vi "Determine Actions.vi"(8 "View":i32[](array[numeric]) caption="View (Team Index, -1: empty)", 9 "Team Index":i32, 10 "Column":i32, 11 "Row":i32) -> (2 "Directions":T1[](array[typedef]), 3 "Actions":T2[](array[typedef]))   [LabVIEW 2015, in "Defenders.lvclass"]
uses:
  Defenders.lvclass
  Type Defs/Action Enum.ctl
  Type Defs/Direction Enum.ctl
  Landscape Global.vi
  Type Defs/SB Type Defs.lvlib
  Common/Common.lvlib
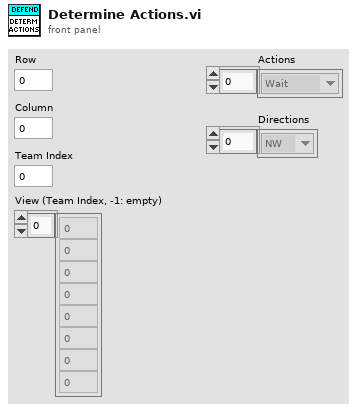
[diagram p1: front panel]
types:
  T1 = typedef "SB Type Defs.lvlib/Direction Enum.ctl" = enum16{"NW", "N", "NE", "E", "SE", "S", "SW", "W"}
  T2 = typedef "SB Type Defs.lvlib/Action Enum.ctl" = enum16{"Wait", "Move", "Attack", "Replicate"}
  T3 = typedef "Defenders.lvclass/Terrain.ctl" = enum16{"Wall", "EnemySighted", "EnemyWall", "Mother", "Move", "StagingArea"}
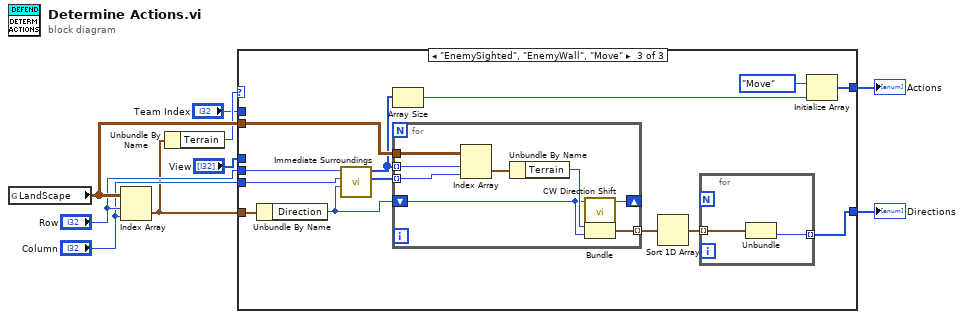
[diagram p0: block diagram]
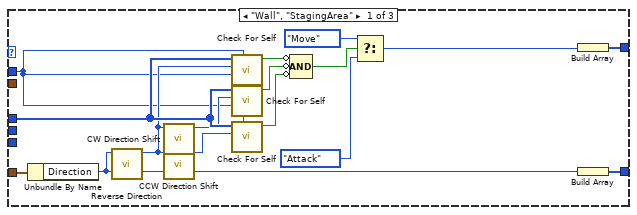
[diagram p2: hidden frame]
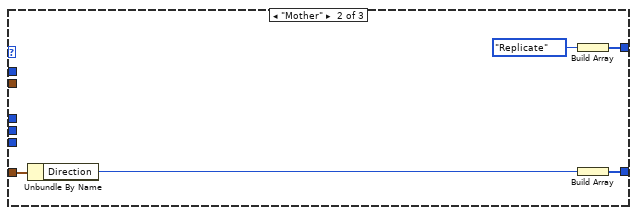
[diagram p3: hidden frame]
diagram:
  n1 = global read "Landscape Global.vi" "LandScape"() -> (w9:cluster{"Terrain":T3, "Direction":T1}[][])
  n2 = Index Array(array=w9, index (row)="Row", index (col)="Column") -> (element=w5:cluster{"Terrain":T3, "Direction":T1})
  n3 = Unbundle By Name(w5) -> ("Terrain"=w6:T3)
  n4 = case shown="\"EnemySighted\", \"EnemyWall\", \"Move\"" w6 {
    tunnel: w9 -> [_ _ w41]
    tunnel: "Row" -> [_ _ w42]
    tunnel: "Column" -> [_ _ w33]
    tunnel: w5 -> [w25 w30 w32]
    tunnel: [w24 w27 w39] -> w4
    tunnel: [w23 w26 w36] -> w3
    tunnel: "View" -> [w16 _ _]
    tunnel: "Team Index" -> [w10 _ _]
    frame "Wall", "StagingArea" {
      n5 = Unbundle By Name(w25) -> ("Direction"=w22:T1)
      n6 = call "Reverse Direction.vi"("Direction in"=w22) -> ("Reverse Direction"=w11:i32)  [unwired: 10 in]
      n7 = call "CW Direction Shift.vi"("Direction"=w11) -> ("Numeric"=w14:i32)  [unwired: 10 in]
      n8 = call "CCW Direction Shift.vi"("Direction"=w11) -> ("Numeric"=w13:i32)  [unwired: 10 in]
      n9 = call "Check For Self.vi"("Team index"=w10, "Direction"=w11, "Map"=w16) -> ("Clear?"=w15:bool)  [unwired: 8 in]
      n10 = call "Check For Self.vi"("Team index"=w10, "Direction"=w14, "Map"=w16) -> ("Clear?"=w17:bool)  [unwired: 8 in]
      n11 = call "Check For Self.vi"("Team index"=w10, "Direction"=w13, "Map"=w16) -> ("Clear?"=w18:bool)  [unwired: 8 in]
      n12 = Compound Arithmetic op=AND(invert w15, invert w17, invert w18) -> (w12:bool)
      n13 = Select(t=Action_Enum."Move" ("Action"), s=w12, f=Action_Enum."Attack" ("Action")) -> (s? t:f=w20:T2)
      n14 = Build Array(w20) -> (w24:T2[])
      n15 = Build Array(w22) -> (w23:T1[])
    }
    frame "Mother" {
      n16 = Unbundle By Name(w30) -> ("Direction"=w28:T1)
      n17 = Build Array(Action_Enum."Replicate" ("Action")) -> (w27:T2[])
      n18 = Build Array(w28) -> (w26:T1[])
    }
    frame "EnemySighted", "EnemyWall", "Move" {
      n19 = Unbundle By Name(w32) -> ("Direction"=w31:T1)
      n20 = call "Immediate Surroundings.vi"("Direction"=w31, "Column"=w33, "Row"=w42) -> ("Columns"=w43:i32[], "Rows"=w35:i32[])  [unwired: 7 in]
      n21 = Array Size(array=w35) -> (size(s)=w34:i32)
      n22 = for {
        tunnel: w41 -> [w53]
        tunnel: w35 -> [w52] mode=indexing
        tunnel: w43 -> [w51] mode=indexing
        tunnel: [w48] -> w38 mode=indexing
        shift-right: [w47] -> _
        shift-left: w31 -> [w46]
        n23 = Index Array(array=w53, index (row)=w52, index (col)=w51) -> (element=w50:cluster{"Terrain":T3, "Direction":T1})
        n24 = Unbundle By Name(w50) -> ("Terrain"=w49:T3)
        n25 = call "CW Direction Shift.vi"("Direction"=w46) -> ("Numeric"=w47:i32)  [unwired: 10 in]
        n26 = Bundle("Terrain"=w49, "Numeric"=w46) -> (w48:cluster{"Terrain":T3, "Numeric":i32})  [unwired: 1 in]
      }
      n27 = Sort 1D Array(array=w38) -> (sorted array=w37:cluster{"Terrain":T3, "Numeric":i32}[])
      n28 = for {
        tunnel: w37 -> [w45] mode=indexing
        tunnel: [w44] -> w36 mode=indexing
        n29 = Unbundle(w45) -> ("Numeric"=w44:i32)  [unwired: 1 out]
      }
      n30 = Initialize Array(Action_Enum."Move" ("Action"), w34) -> (w39:T2[])
    }
  }
  "Actions" <- w4
  "Directions" <- w3
